vi "THETA_3_4.vi"(8 "error in (no error)":errorcluster, 11 "reference in":refnum<class "Manipulator.lvclass">) -> (0 "error out":errorcluster, 3 "reference out":refnum<class "Manipulator.lvclass">)   [LabVIEW 2014, in "Manipulator.lvclass"]
uses:
  Manipulator.lvclass
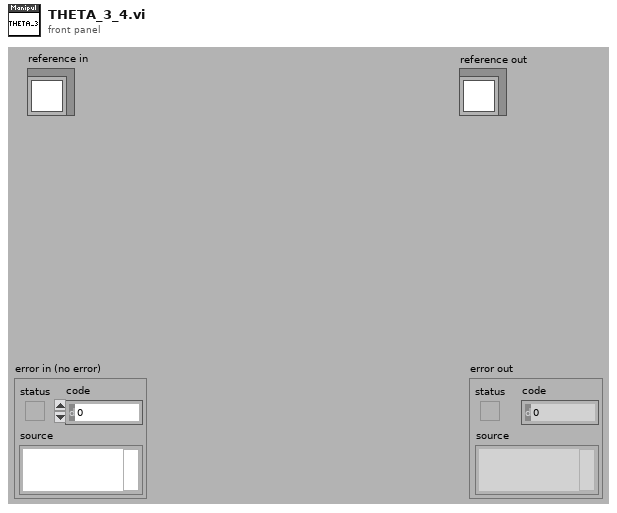
[diagram p1: front panel]
types:
  T1 = typedef "Manipulator.lvclass/ObjectAttributes.ctl" = cluster{"Coordinates":cluster{"X":dbl, "Y":dbl, "Z":dbl}, "Angles":cluster{"THETA_1":dbl, "THETA_2":dbl, "THETA_3":dbl, "THETA_4":dbl, "THETA_5":dbl, "THETA_6":dbl, "THETA_7":dbl, "THETA_8":dbl, "THETA_9":dbl, "THETA_10":dbl}, "Lengths":cluster{"a":dbl, "b":dbl, "c":dbl, "d":dbl, "e":dbl}, "Coordinates of joints":cluster{"A":cluster{"X":dbl, "Y":dbl, "Z":dbl}, "B":cluster{"X":dbl, "Y":dbl, "Z":dbl}, "C":cluster{"X":dbl, "Y":dbl, "Z":dbl}, "D":cluster{"X":dbl, "Y":dbl, "Z":dbl}}}
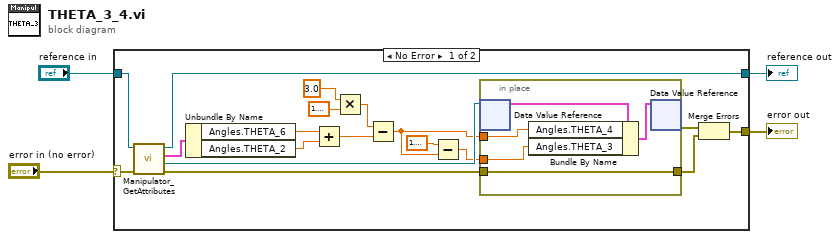
[diagram p0: block diagram]
diagram:
  n1 = case shown="No Error" "error in (no error)" {
    selector: "error in (no error)" -> [w21 w29]
    tunnel: [w17 w29] -> w3
    tunnel: [w18 w28] -> w1
    tunnel: "reference in" -> [w22 w28]
    frame No Error {
      n2 = call "Manipulator_GetAttributes.vi"("error in (no error)"=w21, "reference in"=w22) -> ("error out"=w15:errorcluster, "DataRef"=w16:refnum<data-value>, "Data"=w20:T1, "reference out"=w18:refnum<class "Manipulator.lvclass">)  [unwired: 6 in]
      n3 = Unbundle By Name(w20) -> ("Angles.THETA_6"=w13:dbl, "Angles.THETA_2"=w12:dbl)
      n4 = Add(x=w13, y=w12) -> (x+y=w6:dbl)
      n5 = Multiply(x=3.0, y=1.5707963267948966) -> (x*y=w5:dbl)
      n6 = Subtract(x=w5, y=w6) -> (x-y=w8:dbl)
      n7 = Subtract(x=1.5707963267948966, y=w8) -> (x-y=w7:dbl)
      n8 = in-place {
        in-place-border: w15 -> [w26]
        in-place-border: [w26] -> w14
        in-place-border: w8 -> [w24]
        in-place-border: w7 -> [w23]
        n9 = in-place-dvr #1(w16) -> (w25:T1)  [unwired: 1 out]
        n10 = Bundle By Name(cluster=w25, "Angles.THETA_4"=w24, "Angles.THETA_3"=w23) -> (w27:T1)
        n11 = in-place-dvr #1(w27) -> (w19:errorcluster)  [unwired: 1 out]
      }
      n12 = Merge Errors(w19, w14) -> (w17:errorcluster)
    }
    frame Error {
    }
  }
  "error out" <- w3
  "reference out" <- w1
